vi "Trajectory_Execution_Begin.vi"   [LabVIEW 2019]
uses:
  Trajectory_Execution_Globals.vi
types:
  T1 = typedef "Trajectory_Library.lvlib/TRAJECTORY.ctl" = cluster{"TotalTImeSecs":dbl, "States":T2[]}
  T2 = typedef "Trajectory_Library.lvlib/TRAJ_STATE.ctl" = cluster{"TimeSeconds":dbl, "Velocity":dbl, "Acceleration":dbl, "POSE":T3, "Curvature":dbl}
  T3 = typedef "Trajectory_Library.lvlib/POSE2D.ctl" = cluster{"TRANSLATION":T4, "ROTATION":T5}
  T4 = typedef "Trajectory_Library.lvlib/TRANSLATION2D.ctl" = cluster{"X":dbl, "Y":dbl}
  T5 = typedef "Trajectory_Library.lvlib/ROTATION2D.ctl" = cluster{"VALUE":dbl, "COS":dbl, "SIN":dbl}
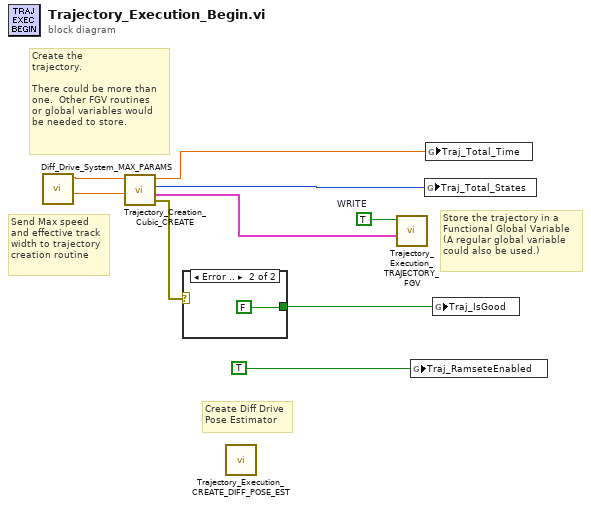
[diagram p0: block diagram]
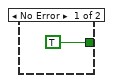
[diagram p2: hidden frame]
diagram:
  w4 = TRUE  # WRITE
  # "Create Diff Drive\nPose Estimator"
  # "Send Max speed\nand effective track\nwidth to trajectory\ncreation routine"
  # "Store the trajectory in a \nFunctional Global Variable\n(A regular global variable\ncould also be used.)"
  # "Create the\ntrajectory.\n\nThere could be more than\none.  Other FGV routines\nor global variables would\nbe needed to store."
  n1 = call "Diff_Drive_System_MAX_PARAMS.vi"() -> ("Effective TrackWidth Ft"=w1:dbl, "Max Speed Ft/Sec"=w2:dbl)  [unwired: 10 in]
  n2 = call "Trajectory_Creation_Cubic_CREATE.vi"("Effective Track Width Ft"=w1, "Max Velocity Ft/Sec"=w2) -> ("Trajectory  creation error"=w9:errorcluster, "Relative Trajectory"=w3:T1, "Trajectory Items"=w7:i32, "TotalTImeSecs"=w8:dbl)  [unwired: 6 in]
  n3 = case shown="Error .." w9 {
    tunnel: [TRUE FALSE] -> w6
    frame No Error {
    }
    frame Error {
    }
  }
  n4 = call "Trajectory_Execution_CREATE_DIFF_POSE_EST.vi"() -> ()  [unwired: 12 in]
  n5 = call "Trajectory_Execution_TRAJECTORY_FGV.vi"("inTRAJECTORY"=w3, "WRITE"=w4) -> ()  [unwired: 9 in, 1 out]
  n6 = global write "Trajectory_Execution_Globals.vi" "Traj_RamseteEnabled"(TRUE) -> ()
  n7 = global write "Trajectory_Execution_Globals.vi" "Traj_Total_States"(w7) -> ()
  n8 = global write "Trajectory_Execution_Globals.vi" "Traj_Total_Time"(w8) -> ()
  n9 = global write "Trajectory_Execution_Globals.vi" "Traj_IsGood"(w6) -> ()
